vi "SwissSPAD Live_Histo Q.vi"(5 "error in (no error)":errorcluster) -> (1 "error out":errorcluster, 2 "SS2 Live Histo Q":refnum<queue>)   [LabVIEW 2021]
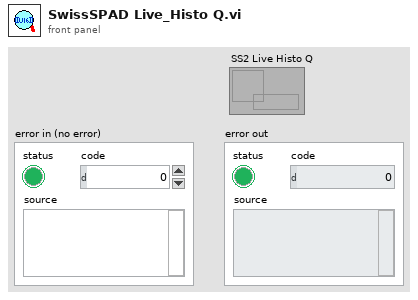
[diagram p1: front panel]
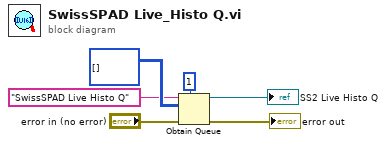
[diagram p0: block diagram]
diagram:
  n1 = Obtain Queue(max queue size (-1, unlimited)=1, name (unnamed)="SwissSPAD Live Histo Q", element data type=u16[][] [], error in (no error)="error in (no error)") -> (queue out=→"SS2 Live Histo Q":refnum<queue>, error out=→"error out":errorcluster)  [unwired: 1 in, 1 out]
